vi "Cal_Settling_Time.vi"(1 "Max Settling Time":dbl=60.0 format="%.2f", 2 "Speed Tweak (m/s)":dbl format="%.2f", 4 "Threshold Value":dbl=0.25 format="%.2f") -> (5 "Required Settling Time":dbl format="%.2f")   [LabVIEW 2018]
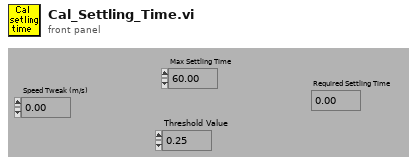
[diagram p1: front panel]
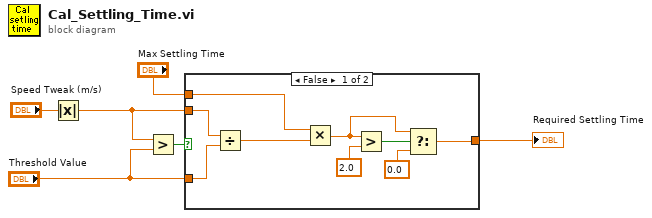
[diagram p0: block diagram]
diagram:
  n1 = Absolute Value(x="Speed Tweak (m/s)") -> (abs(x)=w5:dbl)
  n2 = Greater?(x=w5, y="Threshold Value") -> (0:w6:bool)
  n3 = case shown="False" w6 {
    tunnel: [w7 w16] -> w2
    tunnel: "Max Settling Time" -> [w12 w16]
    tunnel: "Threshold Value" -> [w15 _]
    tunnel: w5 -> [w14 _]
    frame False {
      n4 = Divide(x=w14, y=w15) -> (x/y=w13:dbl)
      n5 = Multiply(x=w12, y=w13) -> (x*y=w9:dbl)
      n6 = Greater?(x=w9, y=2.0) -> (0:w10:bool)
      n7 = Select(t=w9, s=w10, f=0.0) -> (s? t:f=w7:dbl)
    }
    frame True {
    }
  }
  "Required Settling Time" <- w2
